vi "FindMenuItemByTag.vi"(8 "error in (no error)":errorcluster, 10 "Full Tag":string, 11 "NotifyIcon in":refnum<class "MGI_TrayIcon.lvclass">) -> (0 "error out":errorcluster, 2 "Menu Item":refnum<k24>, 3 "NotifyIcon out":refnum<class "MGI_TrayIcon.lvclass">)   [LabVIEW 2016, in "MGI_TrayIcon.lvclass"]
doc: "Searches the menu structure recursively for a menu item with the full tag specified.\n\nAuthored by Derek E. Trepanier\nsupport@mooregoodideas.com\nwww.mooregoodideas.com\n\nCopyright (c) 2012, Moore Good Ideas, Inc.\n\nAll rights reserved.\n\nRedistribution and use in source and binary forms, with or without modification, are permitted provided that the following conditions are met:\n\n * Redistributions of source code must retain the above copyright notice, this list of conditions and the following disclaimer.\n * Redistributions in binary form must reproduce the above copyright notice, this list of conditions and the following disclaimer in the documentation and/or other materials provided with the distribution.\n * Neither the name of Moore Good Ideas, Inc. nor the names of its contributors may be used to endorse or promote products derived from this software without specific prior written permission.\n\nTHIS SOFTWARE IS PROVIDED BY THE COPYRIGHT HOLDERS AND CONTRIBUTORS \"AS IS\" AND ANY EXPRESS OR IMPLIED WARRANTIES, INCLUDING, BUT NOT LIMITED TO, THE IMPLIED WARRANTIES OF MERCHANTABILITY AND FITNESS FOR A PARTICULAR PURPOSE ARE DISCLAIMED. IN NO EVENT SHALL THE COPYRIGHT OWNER OR CONTRIBUTORS BE LIABLE FOR ANY DIRECT, INDIRECT, INCIDENTAL, SPECIAL, EXEMPLARY, OR CONSEQUENTIAL DAMAGES (INCLUDING, BUT NOT LIMITED TO, PROCUREMENT OF SUBSTITUTE GOODS OR SERVICES; LOSS OF USE, DATA, OR PROFITS; OR BUSINESS INTERRUPTION) HOWEVER CAUSED AND ON ANY THEORY OF LIABILITY, WHETHER IN CONTRACT, STRICT LIABILITY, OR TORT (INCLUDING NEGLIGENCE OR OTHERWISE) ARISING IN ANY WAY OUT OF THE USE OF THIS SOFTWARE, EVEN IF ADVISED OF THE POSSIBILITY OF SUCH DAMAGE."
uses:
  <userlib>/_MGI/Menu Building/MenuTypes/TrayIcon/MGI_TrayIcon.lvclass
  System.Windows.Forms
  <userlib>/_MGI/Menu Building/MenuTypes/TrayIcon/MGI_TrayIcon.lvclass/MGI_TrayIcon.ctl
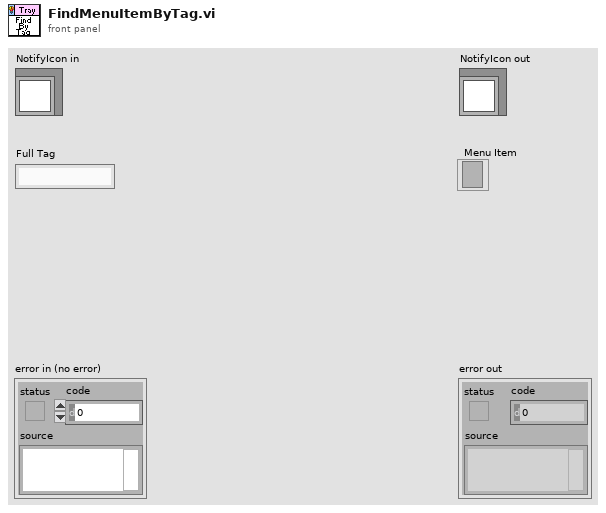
[diagram p1: front panel]
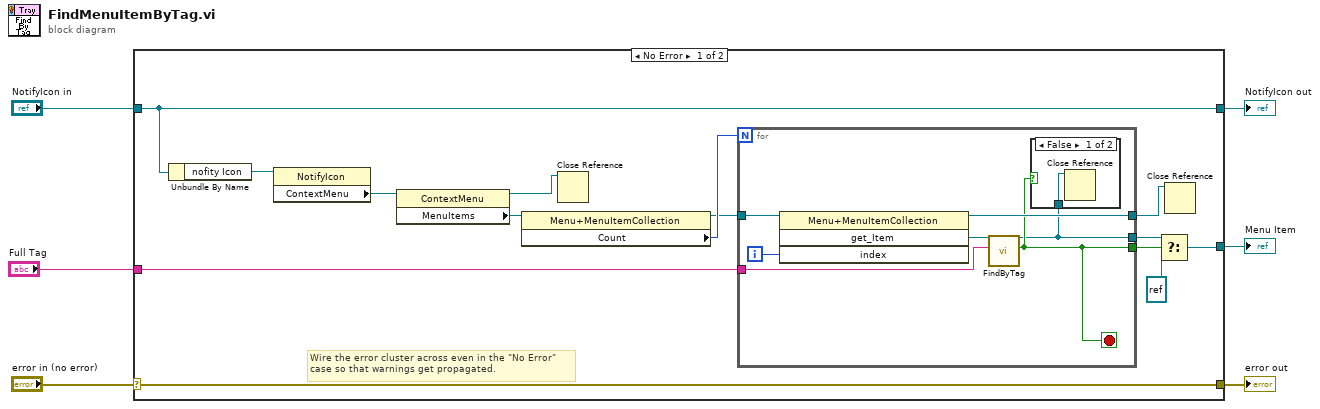
[diagram p0: block diagram]
diagram:
  n1 = case shown="No Error" "error in (no error)" {
    selector: "error in (no error)" -> [w20 w30]
    tunnel: [w20 w30] -> w5
    tunnel: [w19 w29] -> w3
    tunnel: "NotifyIcon in" -> [w19 w29]
    tunnel: "Full Tag" -> [w13 _]
    tunnel: [w11 _] -> w1
    frame No Error {
      # "Wire the error cluster across even in the \"No Error\"\ncase so that warnings get propagated."
      n2 = Unbundle By Name(w19) -> ("nofity Icon"=w18:refnum<k24>)
      n3 = property class="NotifyIcon"(reference=w18) -> ("ContextMenu"=w17:refnum<k24>)  [unwired: 1 in, 2 out]
      n4 = property class="ContextMenu"(reference=w17) -> (reference out=w8:refnum<k24>, "MenuItems"=w16:refnum<k24>)  [unwired: 1 in, 1 out]
      n5 = property class="Menu+MenuItemCollection"(reference=w16) -> (reference out=w14:refnum<k24>, "Count"=w15:i32)  [unwired: 1 in, 1 out]
      n6 = Close Reference(reference=w8) -> ()  [unwired: 1 in, 1 out]
      n7 = for {
        N: w15 -> [_]
        tunnel: w14 -> [w27]
        tunnel: [w21] -> w12
        tunnel: w13 -> [w24]
        tunnel: [w22] -> w9
        tunnel: [w23] -> w7
        i -> [w26]
        stop <- w22 stop-if-true
        n8 = invoke class="Menu+MenuItemCollection" method="get_Item"(reference=w27, "index"=w26) -> (reference out=w23:refnum<k24>, "get_Item"=w25:refnum<k24>)  [unwired: 2 in, 2 out]
        n9 = call <userlib>:"FindByTag.vi"("Full Tag"=w24, "Menu Item In"=w25) -> ("Found?"=w22:bool, "Found Menu Item"=w21:refnum<k24>)  [unwired: 8 in]
        n10 = case shown="False" w22 {
          tunnel: w21 -> [w28 _]
          frame False {
            n11 = Close Reference(reference=w28) -> ()  [unwired: 1 in, 1 out]
          }
          frame True {
          }
        }
      }
      n12 = Select(t=w12, s=w9, f=refnum<k24> refnum) -> (s? t:f=w11:refnum<k24>)
      n13 = Close Reference(reference=w7) -> ()  [unwired: 1 in, 1 out]
    }
    frame Error {
    }
  }
  "error out" <- w5
  "NotifyIcon out" <- w3
  "Menu Item" <- w1
